vi "sub_average_phase.vi"(11 "Input CSI sample":cdb[][][](array[numeric])) -> (3 "Array":dbl[](array[numeric]))   [LabVIEW 2020]
uses:
  <vilib>/Analysis/baseanly.llb/Mean (DBL).vi
  <vilib>/Analysis/NI_AALBase.lvlib
panel:
  out "size(s)":i32[](array[numeric])
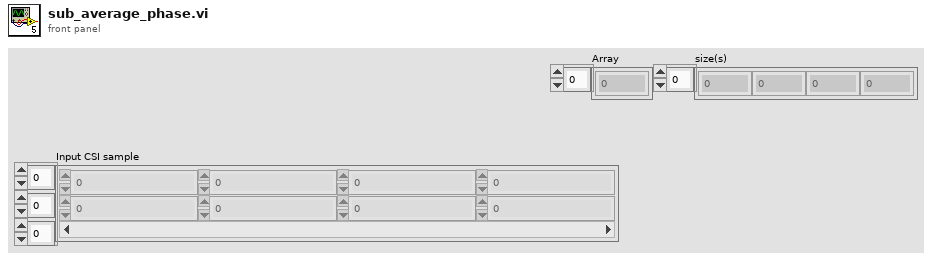
[diagram p1: front panel]
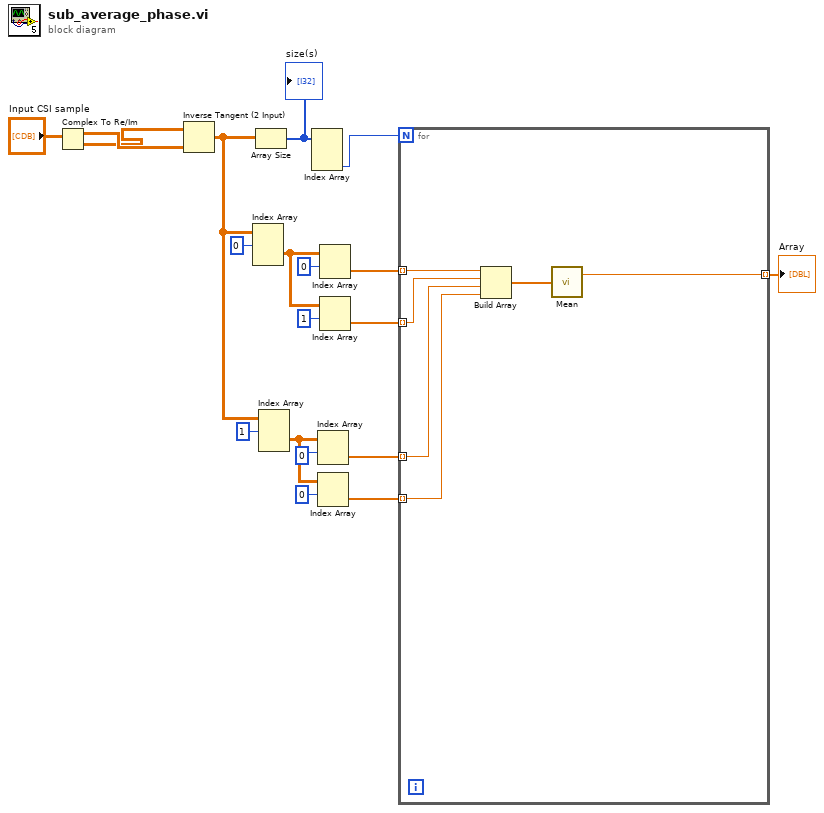
[diagram p0: block diagram]
diagram:
  n1 = Complex To Re/Im(x + iy="Input CSI sample") -> (x=w18:dbl[][][], y=w17:dbl[][][])
  n2 = Inverse Tangent (2 Input)(1:w18, 2:w17) -> (0:w14:dbl[][][])
  n3 = Index Array(array=w14, index (dim 0)=0 ("index (page)")) -> (element=w9:dbl[][])  [unwired: 2 in]
  n4 = Array Size(array=w14) -> (size(s)=w16:i32[])
  "size(s)" <- w16
  n5 = Index Array(array=w14, index (dim 0)=1 ("index (page)")) -> (element=w8:dbl[][])  [unwired: 2 in]
  n6 = Index Array(array=w16) -> (element #3=w15:i32)  [unwired: 3 in, 2 out]
  n7 = Index Array(array=w8, index (row)=0) -> (element=w3:dbl[])  [unwired: 1 in]
  n8 = Index Array(array=w8, index (row)=0) -> (element=w2:dbl[])  [unwired: 1 in]
  n9 = Index Array(array=w9, index (row)=0) -> (element=w5:dbl[])  [unwired: 1 in]
  n10 = Index Array(array=w9, index (row)=1) -> (element=w4:dbl[])  [unwired: 1 in]
  n11 = for {
    N: w15 -> [_]
    tunnel: w5 -> [w25] mode=indexing
    tunnel: w4 -> [w24] mode=indexing
    tunnel: w3 -> [w23] mode=indexing
    tunnel: w2 -> [w22] mode=indexing
    tunnel: [w20] -> w1 mode=indexing
    n12 = Build Array(w25, w24, w23, w22) -> (w21:dbl[])
    n13 = call-poly <vilib>:"Mean.vi"("X"=w21) -> ("mean"=w20:dbl)  [unwired: 1 out]
  }
  "Array" <- w1
